vi "SAOMM-InterpretImageHeader.vi"(7 "ImageHeader":u8[](array[numeric])) -> (1 "ImageWidth":u16, 2 "ImageHeight":u16, 3 "BitPerPixel":u32, 12 "TimeStamp?":u64, 13 "ImageID":u32, 14 "ImageFrameRate":dbl)   [LabVIEW 2019]
panel:
  out "ImageBandWidth":dbl
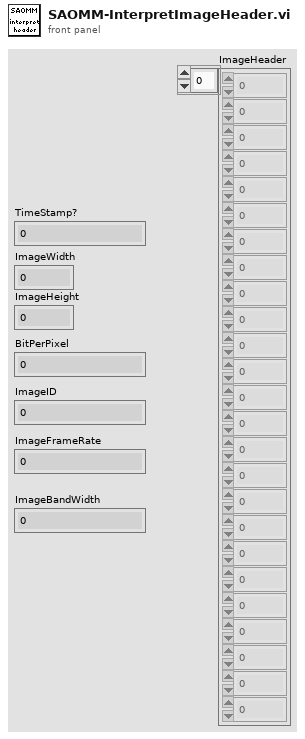
[diagram p1: front panel]
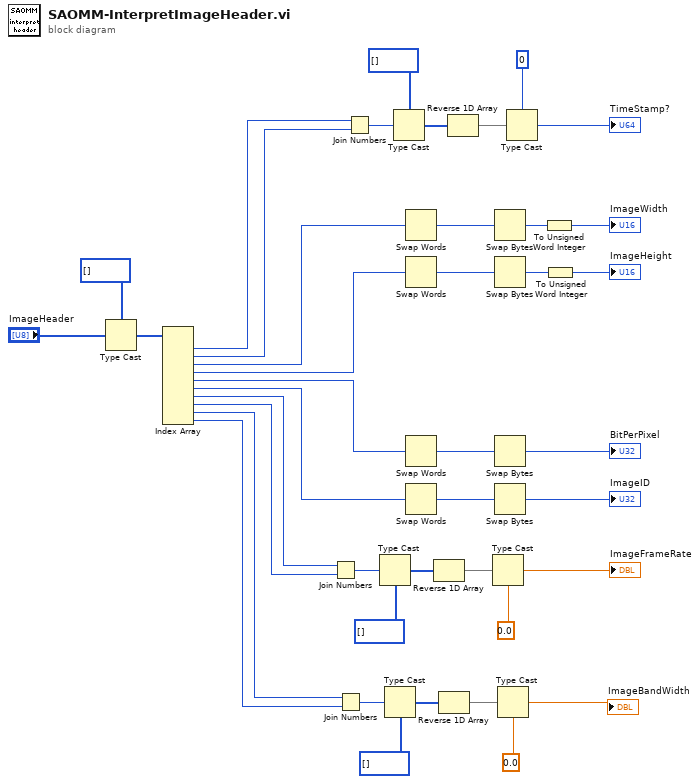
[diagram p0: block diagram]
diagram:
  n1 = Type Cast(type=u32[] [], x="ImageHeader") -> (*(type *) &x=w39:u32[])
  n2 = Index Array(array=w39) -> (element #1=w19:u32, element #2=w20:u32, element #3=w36:u32, element #4=w35:u32, element #5=w30:u32, element #6=w29:u32, element #7=w13:u32, element #8=w12:u32, element #9=w3:u32, element #10=w2:u32)  [unwired: 10 in]
  n3 = Join Numbers(hi=w13, lo=w12) -> ((hi.lo)=w15:u64)
  n4 = Join Numbers(hi=w3, lo=w2) -> ((hi.lo)=w7:u64)
  n5 = Join Numbers(hi=w19, lo=w20) -> ((hi.lo)=w25:u64)
  n6 = Type Cast(type=u8[] [], x=w15) -> (*(type *) &x=w16:u8[])
  n7 = Type Cast(type=u8[] [], x=w7) -> (*(type *) &x=w6:u8[])
  n8 = Type Cast(type=u8[] [], x=w25) -> (*(type *) &x=w24:u8[])
  n9 = Swap Words(1:w36) -> (0:w38:u32)
  n10 = Swap Words(1:w35) -> (0:w37:u32)
  n11 = Swap Words(1:w30) -> (0:w31:u32)
  n12 = Swap Words(1:w29) -> (0:w32:u32)
  n13 = Reverse 1D Array(array=w16) -> (reversed array=w18:u8[])
  n14 = Reverse 1D Array(array=w6) -> (reversed array=w4:u8[])
  n15 = Reverse 1D Array(array=w24) -> (reversed array=w22:u8[])
  n16 = Type Cast(type=0.0, x=w18) -> (*(type *) &x=→"ImageFrameRate":dbl)
  n17 = Swap Bytes(anything=w38) -> (byte swapped=w34:u32)
  n18 = Swap Bytes(anything=w37) -> (byte swapped=w33:u32)
  n19 = Swap Bytes(anything=w31) -> (byte swapped=→"BitPerPixel":u32)
  n20 = Swap Bytes(anything=w32) -> (byte swapped=→"ImageID":u32)
  n21 = Type Cast(type=0.0, x=w4) -> (*(type *) &x=→"ImageBandWidth":dbl)
  n22 = Type Cast(type=u64 0, x=w22) -> (*(type *) &x=→"TimeStamp?":u64)
  n23 = To Unsigned Word Integer(number=w34) -> (unsigned 16bit integer=→"ImageWidth":u16)
  n24 = To Unsigned Word Integer(number=w33) -> (unsigned 16bit integer=→"ImageHeight":u16)
